vi "get_threadRefnum.vi"(8 "error in (no error)":errorcluster, 11 "HGF_ThreadWorker in":refnum<class "HGF_ThreadWorker.lvclass">) -> (0 "error out":errorcluster, 2 "threadRefnum":refnum<vi>, 3 "HGF_ThreadWorker out":refnum<class "HGF_ThreadWorker.lvclass">)   [LabVIEW 2014, in "HGF_BaseClasses.lvlib" / "HGF_ThreadWorker.lvclass"]
uses:
  HGF_ThreadWorker.lvclass
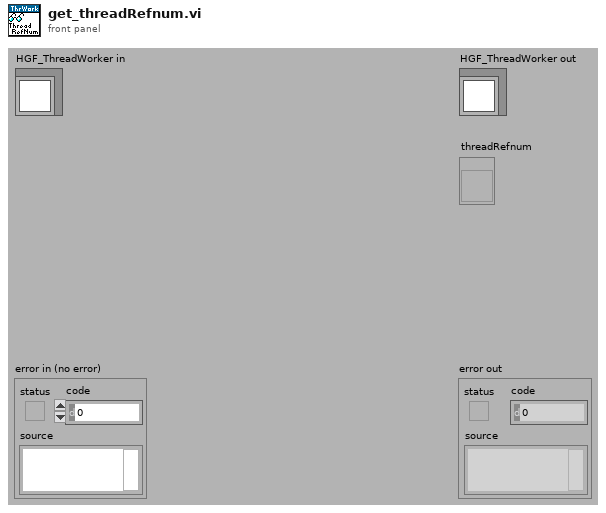
[diagram p1: front panel]
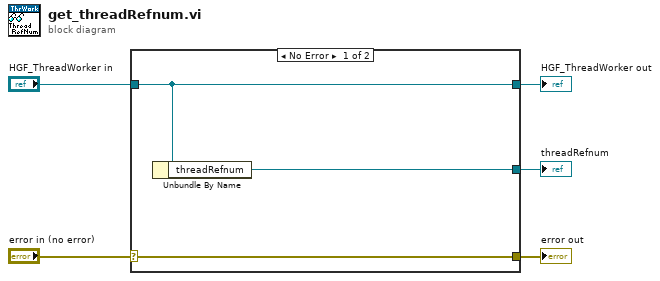
[diagram p0: block diagram]
diagram:
  n1 = case shown="No Error" "error in (no error)" {
    selector: "error in (no error)" -> [w8 w9]
    tunnel: [w8 w9] -> w4
    tunnel: [w7 w10] -> w2
    tunnel: "HGF_ThreadWorker in" -> [w7 w10]
    tunnel: [w6 _] -> w1
    frame No Error {
      n2 = Unbundle By Name(w7) -> ("threadRefnum"=w6:refnum<vi>)
    }
    frame Error {
    }
  }
  "error out" <- w4
  "HGF_ThreadWorker out" <- w2
  "threadRefnum" <- w1
